vi "Check admin.vi"(11 "users in":T1(array[cluster])) -> (1 "admin user?":bool, 2 "name":string, 3 "users out":T1(array[cluster]))   [LabVIEW 2018]
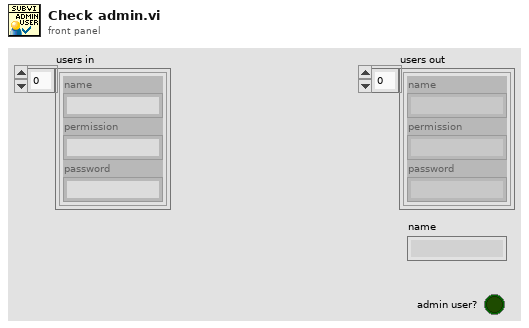
[diagram p1: front panel]
types:
  T1 = cluster{"name":string, "permission":string, "password":string}[]
  T2 = cluster{"name":string, "permission":string, "password":string}
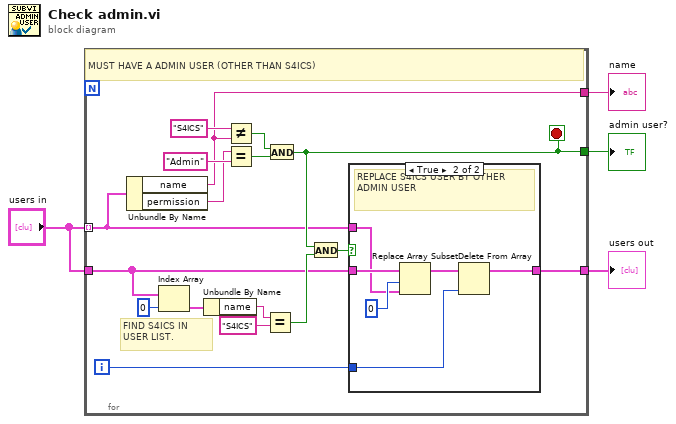
[diagram p0: block diagram]
diagram:
  n1 = for {
    tunnel: [w11] -> w3
    tunnel: "users in" -> [w7] mode=indexing
    tunnel: "users in" -> [w9]
    tunnel: [w6] -> w2
    tunnel: [w5] -> w1
    i -> [w8]
    stop <- w11 stop-if-true
    # "FIND S4ICS IN USER LIST."
    # "MUST HAVE A ADMIN USER (OTHER THAN S4ICS)"
    n2 = Unbundle By Name(w7) -> ("name"=w5:string, "permission"=w17:string)
    n3 = Index Array(array=w9, index=0) -> (element=w15:T2)
    n4 = Unbundle By Name(w15) -> ("name"=w16:string)
    n5 = Not Equal?(x="S4ICS" ("y"), y=w5) -> (x != y?=w19:bool)
    n6 = Equal?(x=w17, y="Admin") -> (x = y?=w18:bool)
    n7 = Equal?(x=w16, y="S4ICS") -> (x = y?=w10:bool)
    n8 = And(x=w19, y=w18) -> (x .and. y?=w11:bool)
    n9 = And(x=w11, y=w10) -> (x .and. y?=w12:bool)
    n10 = case shown="True" w12 {
      tunnel: w9 -> [w22 w28]
      tunnel: w8 -> [_ w25]
      tunnel: w7 -> [_ w26]
      tunnel: [w22 w23] -> w6
      frame False {
      }
      frame True {
        # "REPLACE S4ICS USER BY OTHER\nADMIN USER"
        n11 = Replace Array Subset(array=w28, new element=w26, index=0) -> (w24:T1)
        n12 = Delete From Array(array=w24, index=w25) -> (array with subset deleted=w23:T1)  [unwired: 1 in, 1 out]
      }
    }
  }
  "users out" <- w2
  "admin user?" <- w3
  "name" <- w1
